vi "读取表格.vi"(8 "错误输入":errorcluster, 9 "section":string="报告表格", 10 "Controls[]":refnum<vi>[](array[refnum]), 11 "引用句柄输入":T1 caption="Txt路径") -> (0 "错误输出":errorcluster, 3 "引用句柄输出":T1)   [LabVIEW 2013]
doc: "读取配置文件中的数据，对应显示到表格里"
uses:
  <vilib>/Utility/config.llb/Config Data RefNum.ctl
  <vilib>/Utility/config.llb/Read Key (String).vi
  <vilib>/Utility/config.llb/NI_LVConfig.lvlib
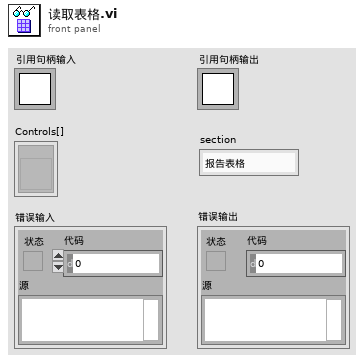
[diagram p1: front panel]
types:
  T1 = typedef "NI_LVConfig.lvlib/Config Data RefNum.ctl" = refnum<k1>
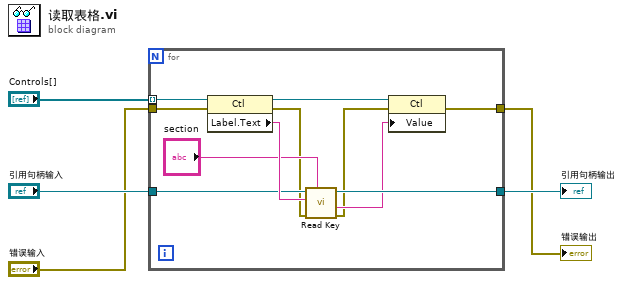
[diagram p0: block diagram]
diagram:
  n1 = for {
    tunnel: "Controls[]" -> [w16] mode=indexing
    tunnel: "引用句柄输入" -> [w12]
    tunnel: [w11] -> w3
    tunnel: "错误输入" -> [w9]
    tunnel: [w6] -> w1
    n2 = property class="Ctl"(reference=w16, error in=w9) -> (reference out=w15:refnum<vi>, error out=w8:errorcluster, "Label.Text"=w14:string)
    n3 = call-poly <vilib>:"Read Key.vi"("section"="section", "error in (no error)"=w8, "key"=w14, "refnum"=w12) -> ("error out"=w7:errorcluster, "value"=w10:string, "refnum out"=w11:T1)  [unwired: 4 in, 1 out]
    n4 = property class="Ctl"(reference=w15, error in=w7, "Value"=w10) -> (error out=w6:errorcluster)  [unwired: 1 out]
  }
  "错误输出" <- w1
  "引用句柄输出" <- w3
